vi "UI.vi"() -> ()   [LabVIEW 2020, in "Modules.lvlib" / "9216.lvclass"]
uses:
  9216.lvclass
  <vilib>/NI VeriStand/Custom Device API/Custom Device Item Ref.ctl
  RSI Module/SubPanel Command.ctl
  RTD Rings for Type and Units.ctl
  RTD Coefficients.ctl
  C:/Users/nitest/Desktop/Git 2020/niveristand-scan-engine-module-libraries/Source/RSI Module/RSI Module.lvclass
  9216.lvclass/9216.ctl
  RSI Module/RSI Module.lvclass
  <vilib>/NI VeriStand/Custom Device API/Custom Device API.lvlib
panel:
  in  "_Measurement Units":u8(ring) items=["Raw Ohms", "Degrees Kelvin", "Degrees Celsius", "Degrees Fahrenheit", "Degrees Rankine"]
  in  "_RTD Type":u8(ring) items=["TCR3851"=1, "TCR3916"=3, "TCR3920"=4, "TCR3911"=5, "TCR3928"=6, "Custom"=0]
  out "Selected Channel Settings Label":string="Selected Channel Settings"
  out "RTD Coefficients Label":string="RTD Coefficients"
  in  "Ro":dbl
  in  "C":dbl
  in  "B":dbl
  in  "A":dbl
  in  "RTD Type":u8(ring) items=["TCR3851"=1, "TCR3916"=3, "TCR3920"=4, "TCR3911"=5, "TCR3928"=6, "Custom"=0]
  in  "Measurement Units":u8(ring) items=["Raw Ohms", "Degrees Kelvin", "Degrees Celsius", "Degrees Fahrenheit", "Degrees Rankine"]
  in  "Channels":i32[](listbox)=[0]
  in  "SubPanel Event":refnum<user-event>
  in  "Header":cluster{"Section Name":string}={"Section Name"="NI 9205 Settings"}
  in  "Conversion Time":u16(ring) items=["200 ms", "2.5 ms"]
  in  "_9216 Config Data":T1={"Conversion Time"=0, "Degree Range"=[], "RTD_Type"=[1], "RTD_A"=[], "RTD_B"=[], "RTD_C"=[], "RTD_Ro"=[]} {"RTD_Type" items=["TCR3851"=1, "TCR3750"=2, "TCR3916"=3, "TCR3920"=4, "TCR3911"=5, "TCR3928"=6, "Custom"=0]; "Degree Range" items=["Raw Ohms", "Degrees Kelvin", "Degrees Celsius", "Degrees Fahrenheit", "Degrees Rankine"]; "Conversion Time" items=["200 ms", "2.5 ms"]}
  in  "Node Ptr":T2 format="%.0x"
  in  "error in (no error)":errorcluster
  out "error out":errorcluster
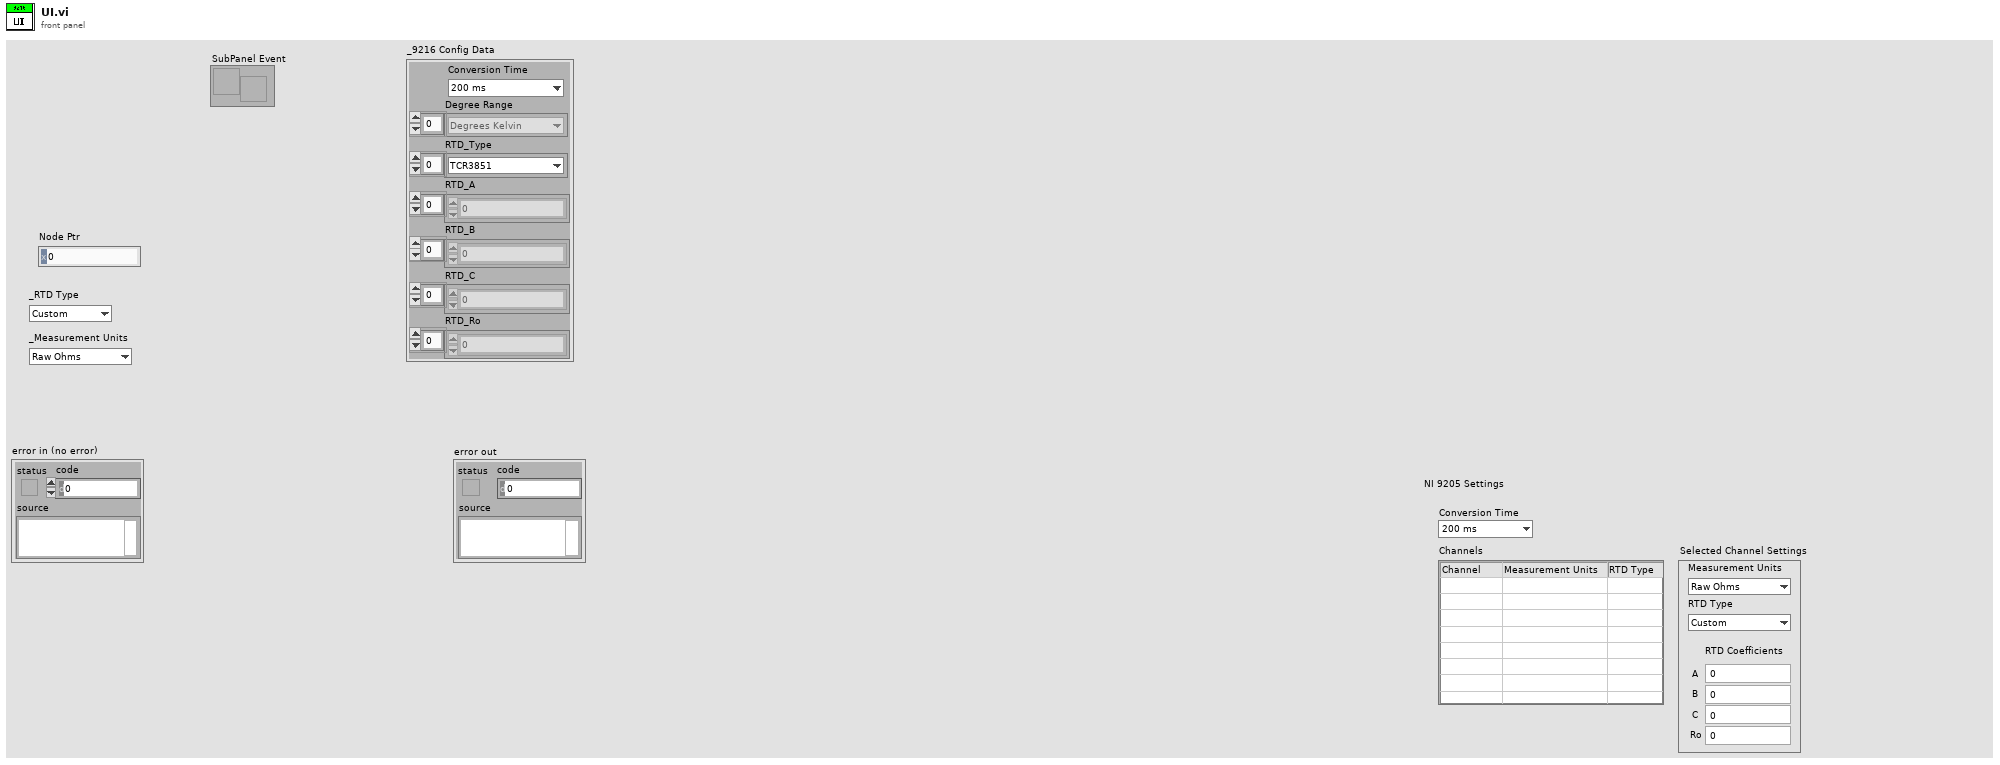
[diagram p1: front panel]
types:
  T1 = cluster{"Conversion Time":u16, "Degree Range":u8[], "RTD_Type":u8[], "RTD_A":dbl[], "RTD_B":dbl[], "RTD_C":dbl[], "RTD_Ro":dbl[]}
  T2 = typedef "Custom Device API.lvlib/Custom Device Item Ref.ctl" = u64
  T3 = typedef "Modules.lvlib/9216.lvclass/RTD Rings for Type and Units.ctl" = cluster{"Type":refnum<vi>, "Units":refnum<vi>}
  T4 = typedef "Modules.lvlib/9216.lvclass/RTD Coefficients.ctl" = cluster{"A":refnum<vi>, "B":refnum<vi>, "C":refnum<vi>, "Ro":refnum<vi>}
  T5 = typedef "Modules.lvlib/RSI Module.lvclass/Channels.ctl" = cluster{"# Input Channels":i32, "# Output Channels":i32, "Channel Type":T6, "Units":string}
  T6 = typedef "Modules.lvlib/RSI Module.lvclass/Channel Type.ctl" = enum16{"Analog", "Digital"}
  T7 = typedef "Modules.lvlib/RSI Module.lvclass/Module Models.ctl" = enum16{"Empty", "NI 9201", "NI 9203", "NI 9205", "NI 9206", "NI 9207", "NI 9208", "NI 9209", "NI 9210", "NI 9211", "NI 9212", "NI 9213", "NI 9214", "NI 9215", "NI 9216", "NI 9217", "NI 9219", "NI 9220", "NI 9221", "NI 9222", "NI 9223", "NI 9224", "NI 9225", "NI 9226", "NI 9227", "NI 9228", "NI 9229", "NI 9233", "NI 9234", "NI 9235", "NI 9236", "NI 9237", "NI 9239", "NI 9242", "NI 9244", "NI 9253", "NI 9263", "NI 9264", "NI 9265", "NI 9266", "NI 9269", "NI 9344", "NI 9350", "NI 9375", "NI 9401", "NI 9402", "NI 9403", "NI 9411", "NI 9421", "NI 9422", "NI 9423", "NI 9425", "NI 9426", "NI 9435", "NI 9436", "NI 9437", "NI 9472", "NI 9474", "NI 9475", "NI 9476", "NI 9477", "NI 9478", "NI 9481", "NI 9482", "NI 9485"}
  T8 = cluster{"Ohm degree range":u32, "RTD type":u32, "RTD user-defined A constant":dbl, "RTD user-defined B constant":dbl, "RTD user-defined C constant":dbl, "RTD user-defined Ro constant":dbl}[]
  T9 = cluster{"Ohm degree range":u32, "RTD type":u32, "RTD user-defined A constant":dbl, "RTD user-defined B constant":dbl, "RTD user-defined C constant":dbl, "RTD user-defined Ro constant":dbl}
  T10 = typedef "LVStringsAndValuesArrayTypeDef_U8.ctl" = cluster{"String":string, "Value":u8}[]
  T11 = typedef "Modules.lvlib/RSI Module.lvclass/SubPanel Command.ctl" = enum16{"Stop"}
  T12 = typedef "Custom Device API.lvlib/Custom Device Channel.ctl" = cluster{"Type":T13, "Units":string, "Default Value":dbl, "Faultable":bool, "Scalable":bool}
  T13 = typedef "Custom Device API.lvlib/Custom Device Channel Type.ctl" = enum16{"Input", "Output"}
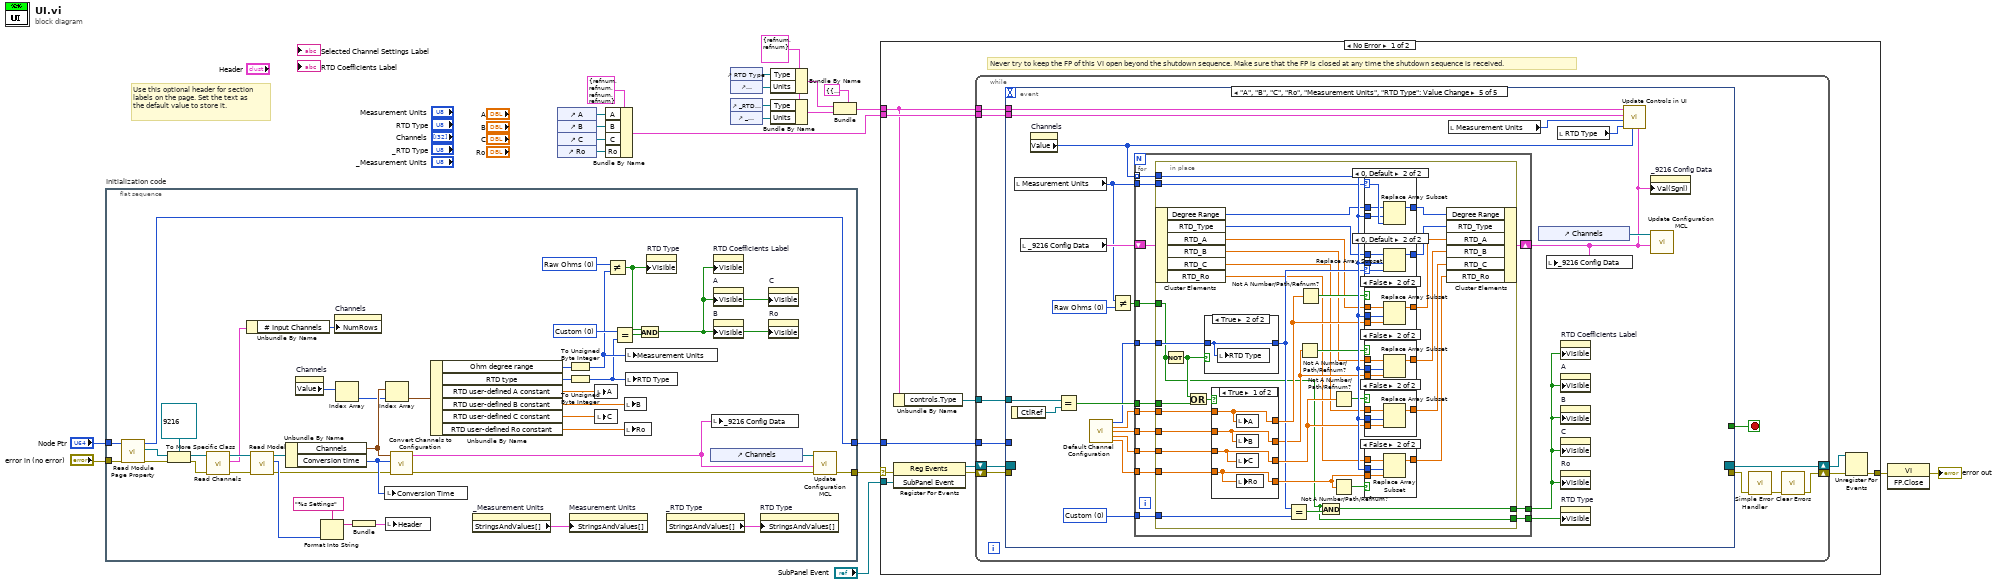
[diagram p0: block diagram]
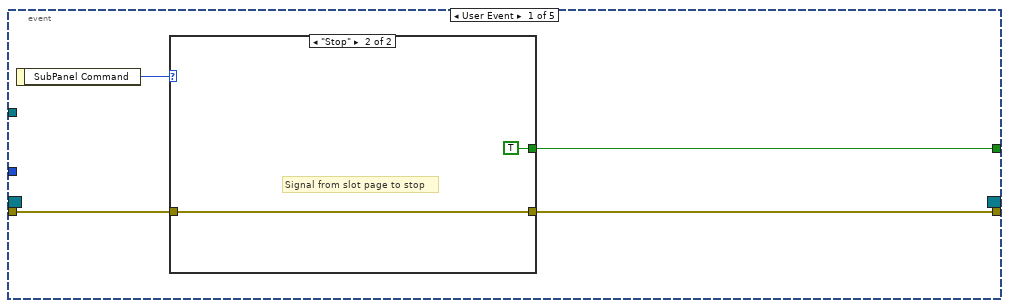
[diagram p2: hidden frame]
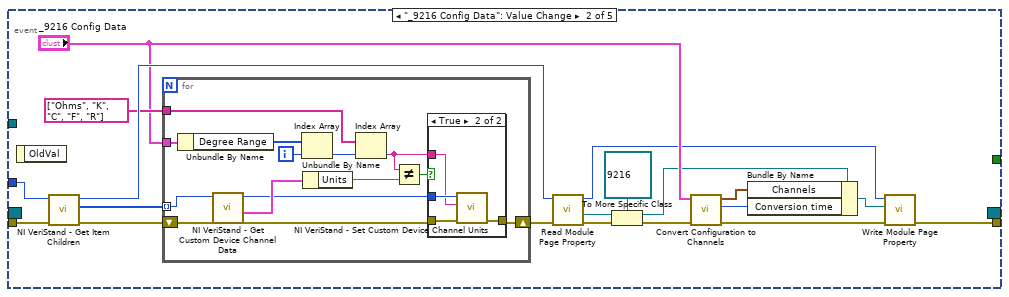
[diagram p4: hidden frame]
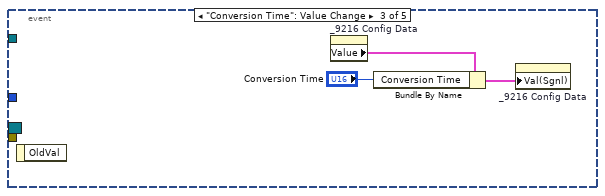
[diagram p6: hidden frame]
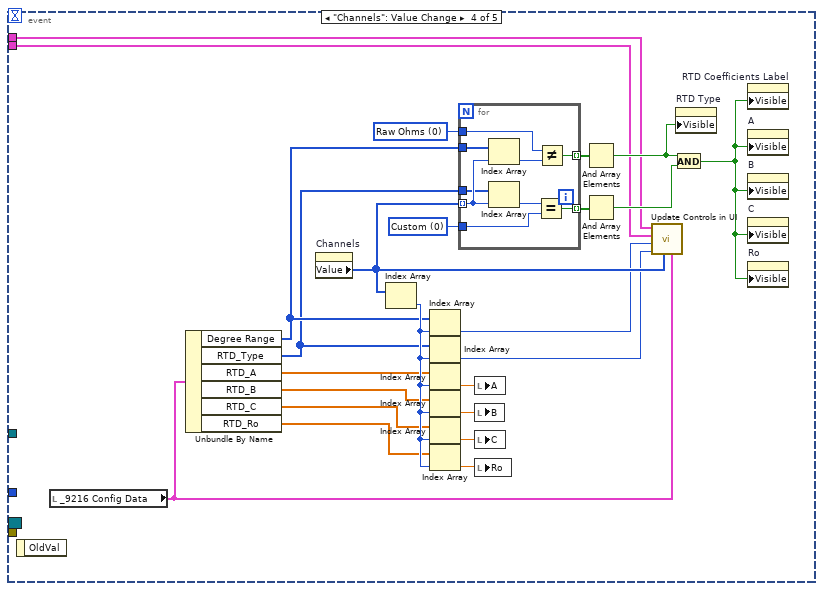
[diagram p7: hidden frame]
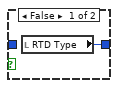
[diagram p8: hidden frame]
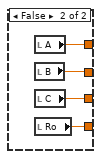
[diagram p9: hidden frame]
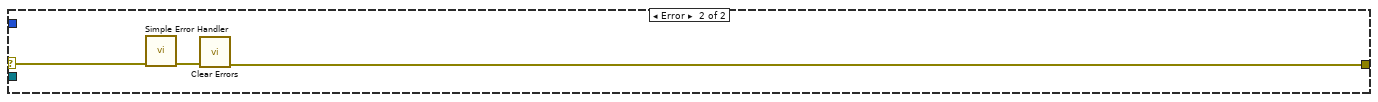
[diagram p16: hidden frame]
diagram:
  w13 = T3 {"Type"=refnum, "Units"=refnum} ("cluster")
  # "Use this optional header for section labels on the page. Set the text as the default value to store it."
  n1 = flat-sequence "Initialization code" {
    tunnel: "error in (no error)" -> [w63]
    tunnel: "Node Ptr" -> [w64]
    tunnel: [w50] -> w16
    tunnel: [w35] -> w19
    frame #0 {
      w47 = u8 0 items=["Raw Ohms", "Degrees Kelvin", "Degrees Celsius", "Degrees Fahrenheit", "Degrees Rankine"] ("Measurement Units")
      w48 = u8 0 items=["TCR3851"=1, "TCR3916"=3, "TCR3920"=4, "TCR3911"=5, "TCR3928"=6, "Custom"=0] ("RTD Type")
      n2 = call "Read Module Page Property.vi"("error in (no error)"=w63, "Node Ptr In"=w64) -> ("error out"=w62:errorcluster, "RSI Module"=w60:refnum<class "RSI Module.lvclass">, "Node Ptr Out"=w35:T2)  [unwired: 7 in]
      n3 = To More Specific Class(target class=refnum<class "9216.lvclass"> refnum ("9205 in"), reference=w60, error in=w62) -> (specific class reference=w41:refnum<class "9216.lvclass">, error out=w39:errorcluster)
      n4 = call "Read Channels.vi"("error in (no error)"=w39, "RSI Module in"=w41) -> ("error out"=w38:errorcluster, "Channels"=w37:T5, "RSI Module out"=w40:refnum<class "9216.lvclass">)  [unwired: 7 in]
      n5 = Unbundle By Name(w37) -> ("# Input Channels"=w36:i32)
      n6 = call "Read Model.vi"("error in (no error)"=w38, "RSI Module in"=w40) -> ("error out"=w53:errorcluster, "Model"=w58:T7, "RSI Module out"=w55:refnum<class "9216.lvclass">)  [unwired: 7 in]
      n7 = Unbundle By Name(w55) -> ("Channels"=w33:T8, "Conversion time"=w54:u16)
      n8 = property on="Channels" class="MCListbox (strict)"() -> ("Value"=w49:i32[])  [unwired: 2 in, 2 out]
      n9 = Format Into String(format string="%s Settings", w58) -> (resulting string=w56:string)  [unwired: 2 in, 1 out]
      n10 = property on="Channels" class="MCListbox (strict)"("NumRows"=w36) -> ()  [unwired: 2 in, 2 out]
      n11 = Index Array(array=w49) -> (element=w31:i32)  [unwired: 1 in]
      n12 = Bundle(w56) -> (w59:cluster{string})  [unwired: 1 in]
      n13 = local write "Conversion Time"(w54) -> ()
      n14 = Index Array(array=w33, index=w31) -> (element=w32:T9)
      n15 = local write "Header"(w59) -> ()
      n16 = call "Convert Channels to Configuration.vi"("error in"=w53, "Conversion time"=w54, "Channels"=w33) -> ("error out"=w51:errorcluster, "_9216 Config Data"=w34:T1)  [unwired: 7 in]
      n17 = Unbundle By Name(w32) -> ("Ohm degree range"=w30:u32, "RTD type"=w28:u32, "RTD user-defined A constant"=w26:dbl, "RTD user-defined B constant"=w25:dbl, "RTD user-defined C constant"=w24:dbl, "RTD user-defined Ro constant"=w23:dbl)
      n18 = property on="_Measurement Units" class="Ring (strict)"() -> ("StringsAndValues[]"=w43:T10)  [unwired: 2 in, 2 out]
      n19 = To Unsigned Byte Integer(number=w30) -> (unsigned 8bit integer=w29:u8)
      n20 = To Unsigned Byte Integer(number=w28) -> (unsigned 8bit integer=w27:u8)
      n21 = property on="Measurement Units" class="Ring (strict)"("StringsAndValues[]"=w43) -> ()  [unwired: 2 in, 2 out]
      n22 = local write "A"(w26) -> ()
      n23 = local write "C"(w24) -> ()
      n24 = Not Equal?(x=w47, y=w29) -> (x != y?=w45:bool)
      n25 = Equal?(x=w48, y=w27) -> (x = y?=w46:bool)
      n26 = local write "B"(w25) -> ()
      n27 = local write "Ro"(w23) -> ()
      n28 = local write "Measurement Units"(w29) -> ()
      n29 = local write "RTD Type"(w27) -> ()
      n30 = And(x=w45, y=w46) -> (x .and. y?=w44:bool)
      n31 = property on="RTD Type" class="Ring (strict)"("Visible"=w45) -> ()  [unwired: 2 in, 2 out]
      n32 = property on="_RTD Type" class="Ring (strict)"() -> ("StringsAndValues[]"=w42:T10)  [unwired: 2 in, 2 out]
      n33 = control-ref of="Channels"() -> (w52:refnum<vi>)
      n34 = local write "_9216 Config Data"(w34) -> ()
      n35 = property on="RTD Coefficients Label" class="Str"("Visible"=w44) -> ()  [unwired: 2 in, 2 out]
      n36 = property on="A" class="DigNum (strict)"("Visible"=w44) -> ()  [unwired: 2 in, 2 out]
      n37 = property on="B" class="DigNum (strict)"("Visible"=w44) -> ()  [unwired: 2 in, 2 out]
      n38 = property on="RTD Type" class="Ring (strict)"("StringsAndValues[]"=w42) -> ()  [unwired: 2 in, 2 out]
      n39 = property on="C" class="DigNum (strict)"("Visible"=w44) -> ()  [unwired: 2 in, 2 out]
      n40 = property on="Ro" class="DigNum (strict)"("Visible"=w44) -> ()  [unwired: 2 in, 2 out]
      n41 = call "Update Configuration MCL.vi"("error in"=w51, "_9216 Config"=w34, "_Channel Refnum"=w52) -> ("error out"=w50:errorcluster)  [unwired: 6 in]
    }
  }
  n42 = control-ref of="A"() -> (w8:refnum<vi>)
  n43 = control-ref of="B"() -> (w7:refnum<vi>)
  n44 = control-ref of="C"() -> (w6:refnum<vi>)
  n45 = control-ref of="Ro"() -> (w5:refnum<vi>)
  n46 = Bundle By Name(cluster=T4 {"A"=refnum, "B"=refnum, "C"=refnum, "Ro"=refnum} ("RTD coefficients"), "A"=w8, "B"=w7, "C"=w6, "Ro"=w5) -> (w2:T4)
  n47 = control-ref of="RTD Type"() -> (w15:refnum<vi>)
  n48 = control-ref of="Measurement Units"() -> (w14:refnum<vi>)
  n49 = control-ref of="_RTD Type"() -> (w12:refnum<vi>)
  n50 = control-ref of="_Measurement Units"() -> (w11:refnum<vi>)
  n51 = Bundle By Name(cluster=w13, "Type"=w15, "Units"=w14) -> (w10:T3)
  n52 = Bundle By Name(cluster=w13, "Type"=w12, "Units"=w11) -> (w9:T3)
  n53 = Bundle(cluster=cluster{"controls":T3, "typedefs":T3} {"controls"={"Type"=refnum, "Units"=refnum}, "typedefs"={"Type"=refnum, "Units"=refnum}}, "controls"=w10, "typedefs"=w9) -> (w3:cluster{"controls":T3, "typedefs":T3})
  n54 = case shown="No Error" w16 {
    selector: w16 -> [w69 w281]
    tunnel: [w73 w279] -> w22
    tunnel: w19 -> [w70 _]
    tunnel: "SubPanel Event" -> [w68 _]
    tunnel: w3 -> [w66 _]
    tunnel: w2 -> [w67 _]
    frame No Error {
      # "Never try to keep the FP of this VI open beyond the shutdown sequence. Make sure that the FP is closed at any time the shutdown sequence is received."
      n55 = Unbundle By Name(w66) -> ("controls.Type"=w65:refnum<vi>)
      n56 = register-events(error in=w69, w68) -> (reference out=w71:refnum<event-registration>, error out=w72:errorcluster)  [unwired: 1 in]
      n57 = while {
        tunnel: w70 -> [w82]
        shift-right: [w79] -> w74
        shift-left: w72 -> [w85]
        shift-right: [w86] -> w75
        shift-left: w71 -> [w84]
        tunnel: w66 -> [w78]
        tunnel: w67 -> [w77]
        tunnel: w65 -> [w76]
        stop <- w83 stop-if-true
        n58 = event shown="[4] \"A\", \"B\", \"C\", \"Ro\", \"Measurement Units\", \"RTD Type\": Value Change" {
          selector: w84 -> [_ _ _ _ _]
          dyn-events: [_ _ _ _ _] -> w86
          timeout: _ -> [_ _ _ _ _]
          tunnel: w85 -> [w89 w103 _ _ _]
          tunnel: [w88 _ _ _ _] -> w83
          tunnel: [w87 w109 _ _ _] -> w81
          tunnel: w82 -> [_ w104 _ _ _]
          tunnel: w78 -> [_ _ _ w138 w183]
          tunnel: w77 -> [_ _ _ w136 w182]
          tunnel: w76 -> [_ _ _ _ w181]
          event User Event {
            n59 = event-data() -> ("SubPanel Command"=w90:T11)  [unwired: 1 out]
            n60 = case shown="\"Stop\"" w90 {
              tunnel: w89 -> [w91 w92]
              tunnel: [w91 w92] -> w87
              tunnel: [_ TRUE] -> w88
              frame Default {
              }
              frame "Stop" {
                # "Signal from slot page to stop"
              }
            }
          }
          event "_9216 Config Data": Value Change {
            n61 = event-data() -> ()  [unwired: 2 out]
            n62 = call <vilib>:"NI VeriStand - Get Item Children.vi"("error in (no error)"=w103, "Item Ref in"=w104) -> ("error out"=w102:errorcluster, "Child Refs"=w101:T2[], "Item Ref out"=w100:T2)  [unwired: 6 in, 1 out]
            n63 = for {
              tunnel: w101 -> [w118] mode=indexing
              shift-right: [w119] -> w99
              shift-left: w102 -> [w121]
              tunnel: "_9216 Config Data" -> [w126]
              tunnel: string[] ["Ohms", "K", "C", "F", "R"] -> [w125]
              i -> [w115]
              n64 = Unbundle By Name(w126) -> ("Degree Range"=w116:u8[])
              n65 = call <vilib>:"NI VeriStand - Get Custom Device Channel Data.vi"("error in (no error)"=w121, "Channel Ref in"=w118) -> ("error out"=w120:errorcluster, "Channel"=w123:T12, "Channel Ref out"=w117:T2)  [unwired: 4 in, 3 out]
              n66 = Index Array(array=w116, index=w115) -> (element=w114:u8)
              n67 = Unbundle By Name(w123) -> ("Units"=w122:string)
              n68 = Index Array(array=w125, index=w114) -> (element=w113:string)
              n69 = Not Equal?(x=w113, y=w122) -> (x != y?=w124:bool)
              n70 = case shown="True" w124 {
                tunnel: w117 -> [_ w131]
                tunnel: w113 -> [_ w130]
                tunnel: w120 -> [w127 w129]
                tunnel: [w127 w128] -> w119
                frame False {
                }
                frame True {
                  n71 = call <vilib>:"NI VeriStand - Set Custom Device Channel Units.vi"("error in (no error)"=w129, "Units"=w130, "Channel Ref in"=w131) -> ("error out"=w128:errorcluster)  [unwired: 7 in, 1 out]
                }
              }
            }
            n72 = call "Read Module Page Property.vi"("error in (no error)"=w99, "Node Ptr In"=w100) -> ("error out"=w110:errorcluster, "RSI Module"=w111:refnum<class "RSI Module.lvclass">, "Node Ptr Out"=w95:T2)  [unwired: 7 in]
            n73 = To More Specific Class(target class=refnum<class "9216.lvclass"> refnum ("9216"), reference=w111, error in=w110) -> (specific class reference=w94:refnum<class "9216.lvclass">, error out=w107:errorcluster)
            n74 = call "Convert Configuration to Channels.vi"("error in"=w107, "_9216 Config Data"="_9216 Config Data") -> ("error out"=w106:errorcluster, "Conversion Time"=w105:u16, "Channels"=w108:T8)  [unwired: 7 in]
            n75 = Bundle By Name(cluster=w94, "Channels"=w108, "Conversion time"=w105) -> (w96:refnum<class "9216.lvclass">)
            n76 = call "Write Module Page Property.vi"("error in (no error)"=w106, "RSI Module"=w96, "Node Ptr In"=w95) -> ("error out"=w109:errorcluster)  [unwired: 6 in, 2 out]
          }
          event "Conversion Time": Value Change {
            n77 = event-data() -> ()  [unwired: 2 out]
            n78 = property on="_9216 Config Data" class="Clust (strict)"() -> ("Value"=w134:T1)  [unwired: 2 in, 2 out]
            n79 = Bundle By Name(cluster=w134, "Conversion Time"="Conversion Time") -> (w132:T1)
            n80 = property on="_9216 Config Data" class="Clust (strict)"("Val(Sgnl)"=w132) -> ()  [unwired: 2 in, 2 out]
          }
          event "Channels": Value Change {
            w135 = u8 0 items=["TCR3851"=1, "TCR3750"=2, "TCR3916"=3, "TCR3920"=4, "TCR3911"=5, "TCR3928"=6, "Custom"=0] ("RTD Type")
            w137 = u8 0 items=["Raw Ohms", "Degrees Kelvin", "Degrees Celsius", "Degrees Fahrenheit", "Degrees Rankine"] ("Measurement Units")
            n81 = event-data() -> ()  [unwired: 2 out]
            n82 = local read "_9216 Config Data"() -> (w142:T1)
            n83 = Unbundle By Name(w142) -> ("Degree Range"=w149:u8[], "RTD_Type"=w148:u8[], "RTD_A"=w150:dbl[], "RTD_B"=w151:dbl[], "RTD_C"=w152:dbl[], "RTD_Ro"=w153:dbl[])
            n84 = property on="Channels" class="MCListbox (strict)"() -> ("Value"=w141:i32[])  [unwired: 2 in, 2 out]
            n85 = Index Array(array=w141) -> (element=w154:i32)  [unwired: 1 in]
            n86 = Index Array(array=w149, index=w154) -> (element=w139:u8)
            n87 = Index Array(array=w148, index=w154) -> (element=w140:u8)
            n88 = Index Array(array=w150, index=w154) -> (element=w158:dbl)
            n89 = Index Array(array=w151, index=w154) -> (element=w157:dbl)
            n90 = Index Array(array=w152, index=w154) -> (element=w156:dbl)
            n91 = Index Array(array=w153, index=w154) -> (element=w155:dbl)
            n92 = for {
              tunnel: w141 -> [w167] mode=indexing
              tunnel: w149 -> [w166]
              tunnel: w148 -> [w165]
              tunnel: [w162] -> w147 mode=indexing
              tunnel: [w161] -> w146 mode=indexing
              tunnel: w137 -> [w160]
              tunnel: w135 -> [w159]
              n93 = Index Array(array=w166, index=w167) -> (element=w164:u8)
              n94 = Index Array(array=w165, index=w167) -> (element=w163:u8)
              n95 = Equal?(x=w163, y=w159) -> (x = y?=w161:bool)
              n96 = Not Equal?(x=w160, y=w164) -> (x != y?=w162:bool)
            }
            n97 = local write "A"(w158) -> ()
            n98 = local write "B"(w157) -> ()
            n99 = local write "C"(w156) -> ()
            n100 = local write "Ro"(w155) -> ()
            n101 = And Array Elements(Boolean array=w147) -> (logical AND=w144:bool)
            n102 = And Array Elements(Boolean array=w146) -> (logical AND=w145:bool)
            n103 = call "Update Controls in UI.vi"("9216 Config"=w142, "Values"=w141, "RTD Type"=w140, "Units"=w139, "RTD coefficients"=w136, "RTD types and units controls"=w138) -> ()  [unwired: 6 in]
            n104 = And(x=w144, y=w145) -> (x .and. y?=w143:bool)
            n105 = property on="RTD Type" class="Ring (strict)"("Visible"=w144) -> ()  [unwired: 2 in, 2 out]
            n106 = property on="RTD Coefficients Label" class="Str"("Visible"=w143) -> ()  [unwired: 2 in, 2 out]
            n107 = property on="A" class="DigNum (strict)"("Visible"=w143) -> ()  [unwired: 2 in, 2 out]
            n108 = property on="B" class="DigNum (strict)"("Visible"=w143) -> ()  [unwired: 2 in, 2 out]
            n109 = property on="C" class="DigNum (strict)"("Visible"=w143) -> ()  [unwired: 2 in, 2 out]
            n110 = property on="Ro" class="DigNum (strict)"("Visible"=w143) -> ()  [unwired: 2 in, 2 out]
          }
          event "A", "B", "C", "Ro", "Measurement Units", "RTD Type": Value Change {
            w168 = u8 0 items=["TCR3851"=1, "TCR3916"=3, "TCR3920"=4, "TCR3911"=5, "TCR3928"=6, "Custom"=0] ("RTD Type")
            w172 = u8 0 items=["Raw Ohms", "Degrees Kelvin", "Degrees Celsius", "Degrees Fahrenheit", "Degrees Rankine"] ("Measurement Units")
            n111 = event-data() -> ("CtlRef"=w186:refnum<vi>)  [unwired: 1 out]
            n112 = local read "Measurement Units"() -> (w171:u8)
            n113 = local read "_9216 Config Data"() -> (w178:T1)
            n114 = property on="Channels" class="MCListbox (strict)"() -> ("Value"=w187:i32[])  [unwired: 2 in, 2 out]
            n115 = Equal?(x=w181, y=w186) -> (x = y?=w185:bool)
            n116 = call "Default Channel Configuration.vi"() -> ("RTD Types"=w177:u8, "RTD_A"=w176:dbl, "RTD_B"=w175:dbl, "RTD_C"=w174:dbl, "RTD_Ro"=w173:dbl)  [unwired: 9 in, 2 out]
            n117 = Not Equal?(x=w171, y=w172) -> (x != y?=w170:bool)
            n118 = for {
              tunnel: w187 -> [w202] mode=indexing
              tunnel: w185 -> [w203]
              tunnel: [w201] -> w180
              shift-right: [w191] -> w179
              shift-left: w178 -> [w192]
              tunnel: w177 -> [w200]
              tunnel: w176 -> [w199]
              tunnel: w175 -> [w198]
              tunnel: w174 -> [w197]
              tunnel: w173 -> [w196]
              tunnel: w170 -> [w194]
              tunnel: w171 -> [w195]
              tunnel: [w190] -> w169
              tunnel: w168 -> [w193]
              n119 = in-place {
                in-place-border: w203 -> [w238]
                in-place-border: w202 -> [w236]
                in-place-border: [w225] -> w201
                in-place-border: w200 -> [w224]
                in-place-border: w199 -> [w223]
                in-place-border: w198 -> [w222]
                in-place-border: w197 -> [w221]
                in-place-border: w196 -> [w220]
                in-place-border: w195 -> [w219]
                in-place-border: w194 -> [w204]
                in-place-border: w193 -> [w218]
                in-place-border: [w204] -> w190
                n120 = in-place-cluster #1(w192) -> ("Degree Range"=w211:u8[], "RTD_Type"=w212:u8[], "RTD_A"=w213:dbl[], "RTD_B"=w214:dbl[], "RTD_C"=w215:dbl[], "RTD_Ro"=w216:dbl[])
                n121 = Not(x=w204) -> (.not. x?=w228:bool)
                n122 = Or(x=w228, y=w238) -> (x .or. y?=w237:bool)
                n123 = case shown="True" w228 {
                  tunnel: [w239 w240] -> w227
                  tunnel: w224 -> [_ w240]
                  frame False {
                    n124 = local read "RTD Type"() -> (w239:u8)
                  }
                  frame True {
                    n125 = local write "RTD Type"(w240) -> ()
                  }
                }
                n126 = case shown="True" w237 {
                  tunnel: w223 -> [w244 _]
                  tunnel: w222 -> [w243 _]
                  tunnel: w221 -> [w242 _]
                  tunnel: w220 -> [w241 _]
                  tunnel: [w244 w248] -> w230
                  tunnel: [w243 w247] -> w217
                  tunnel: [w242 w246] -> w232
                  tunnel: [w241 w245] -> w234
                  frame True {
                    n127 = local write "A"(w244) -> ()
                    n128 = local write "B"(w243) -> ()
                    n129 = local write "C"(w242) -> ()
                    n130 = local write "Ro"(w241) -> ()
                  }
                  frame False {
                    n131 = local read "A"() -> (w248:dbl)
                    n132 = local read "B"() -> (w247:dbl)
                    n133 = local read "C"() -> (w246:dbl)
                    n134 = local read "Ro"() -> (w245:dbl)
                  }
                }
                n135 = Equal?(x=w227, y=w218) -> (x = y?=w226:bool)
                n136 = Not A Number/Path/Refnum?(number/path/refnum=w217) -> (NaN/Path/Refnum?=w231:bool)
                n137 = Not A Number/Path/Refnum?(number/path/refnum=w230) -> (NaN/Path/Refnum?=w229:bool)
                n138 = And(x=w204, y=w226) -> (x .and. y?=w225:bool)
                n139 = Not A Number/Path/Refnum?(number/path/refnum=w232) -> (NaN/Path/Refnum?=w233:bool)
                n140 = Not A Number/Path/Refnum?(number/path/refnum=w234) -> (NaN/Path/Refnum?=w235:bool)
                n141 = case shown="0, Default" w219 {
                  selector: w219 -> [_ w277]
                  tunnel: [w274 w278] -> w210
                  tunnel: w211 -> [w274 w276]
                  tunnel: w236 -> [_ w275]
                  frame 99 {
                  }
                  frame 0, Default {
                    n142 = Replace Array Subset(array=w276, new element=w277, index=w275) -> (w278:u8[])
                  }
                }
                n143 = case shown="0, Default" w227 {
                  selector: w227 -> [_ w272]
                  tunnel: [w269 w273] -> w209
                  tunnel: w212 -> [w269 w271]
                  tunnel: w236 -> [_ w270]
                  frame 99 {
                  }
                  frame 0, Default {
                    n144 = Replace Array Subset(array=w271, new element=w272, index=w270) -> (w273:u8[])
                  }
                }
                n145 = case shown="False" w229 {
                  tunnel: [w264 w268] -> w208
                  tunnel: w213 -> [w264 w267]
                  tunnel: w236 -> [_ w266]
                  tunnel: w230 -> [_ w265]
                  frame True {
                  }
                  frame False {
                    n146 = Replace Array Subset(array=w267, new element=w265, index=w266) -> (w268:dbl[])
                  }
                }
                n147 = case shown="False" w231 {
                  tunnel: [w259 w263] -> w207
                  tunnel: w214 -> [w259 w262]
                  tunnel: w236 -> [_ w261]
                  tunnel: w217 -> [_ w260]
                  frame True {
                  }
                  frame False {
                    n148 = Replace Array Subset(array=w262, new element=w260, index=w261) -> (w263:dbl[])
                  }
                }
                n149 = case shown="False" w233 {
                  tunnel: [w254 w258] -> w206
                  tunnel: w215 -> [w254 w257]
                  tunnel: w236 -> [_ w256]
                  tunnel: w232 -> [_ w255]
                  frame True {
                  }
                  frame False {
                    n150 = Replace Array Subset(array=w257, new element=w255, index=w256) -> (w258:dbl[])
                  }
                }
                n151 = case shown="False" w235 {
                  tunnel: [w249 w253] -> w205
                  tunnel: w216 -> [w249 w252]
                  tunnel: w236 -> [_ w251]
                  tunnel: w234 -> [_ w250]
                  frame True {
                  }
                  frame False {
                    n152 = Replace Array Subset(array=w252, new element=w250, index=w251) -> (w253:dbl[])
                  }
                }
                n153 = in-place-cluster #1("Degree Range"=w210, "RTD_Type"=w209, "RTD_A"=w208, "RTD_B"=w207, "RTD_C"=w206, "RTD_Ro"=w205) -> (w191:T1)
              }
            }
            n154 = local read "Measurement Units"() -> (w189:u8)
            n155 = control-ref of="Channels"() -> (w184:refnum<vi>)
            n156 = local write "_9216 Config Data"(w179) -> ()
            n157 = local read "RTD Type"() -> (w188:u8)
            n158 = property on="RTD Coefficients Label" class="Str"("Visible"=w180) -> ()  [unwired: 2 in, 2 out]
            n159 = property on="A" class="DigNum (strict)"("Visible"=w180) -> ()  [unwired: 2 in, 2 out]
            n160 = property on="B" class="DigNum (strict)"("Visible"=w180) -> ()  [unwired: 2 in, 2 out]
            n161 = property on="C" class="DigNum (strict)"("Visible"=w180) -> ()  [unwired: 2 in, 2 out]
            n162 = property on="Ro" class="DigNum (strict)"("Visible"=w180) -> ()  [unwired: 2 in, 2 out]
            n163 = property on="RTD Type" class="Ring (strict)"("Visible"=w169) -> ()  [unwired: 2 in, 2 out]
            n164 = call "Update Controls in UI.vi"("9216 Config"=w179, "Values"=w187, "RTD Type"=w188, "Units"=w189, "RTD coefficients"=w182, "RTD types and units controls"=w183) -> ()  [unwired: 6 in]
            n165 = property on="_9216 Config Data" class="Clust (strict)"("Val(Sgnl)"=w179) -> ()  [unwired: 2 in, 2 out]
            n166 = call "Update Configuration MCL.vi"("_9216 Config"=w179, "_Channel Refnum"=w184) -> ()  [unwired: 7 in, 1 out]
          }
        }
        n167 = call <vilib>:"Simple Error Handler.vi"("error in (no error)"=w81) -> ("error out"=w80:errorcluster)  [unwired: 1 in, 7 out]
        n168 = call <vilib>:"Clear Errors.vi"("error in (no error)"=w80) -> ("error out"=w79:errorcluster)  [unwired: 1 in, 5 out]
      }
      n169 = Unregister For Events(event registration refnum=w75, error in=w74) -> (error out=w73:errorcluster)
    }
    frame Error {
      n170 = call <vilib>:"Simple Error Handler.vi"("error in (no error)"=w281) -> ("error out"=w280:errorcluster)  [unwired: 1 in, 7 out]
      n171 = call <vilib>:"Clear Errors.vi"("error in (no error)"=w280) -> ("error out"=w279:errorcluster)  [unwired: 1 in, 5 out]
    }
  }
  n172 = invoke class="VI" method="FP.Close"(error in=w22) -> (error out=→"error out":errorcluster)  [unwired: 2 in, 2 out]
